vi "opencvDisplayImageTest.vi"() -> ()   [LabVIEW 2017]
uses:
  globalUtilities.vi
panel:
  out "x-y":dbl format="%.9f"
  in  "stop 4":bool
  out "Intensity Graph":u16[][](graph)
  in  "stop 3":bool
  # "Arrays work only if they have size >1 (2 is fine). Dunno why."
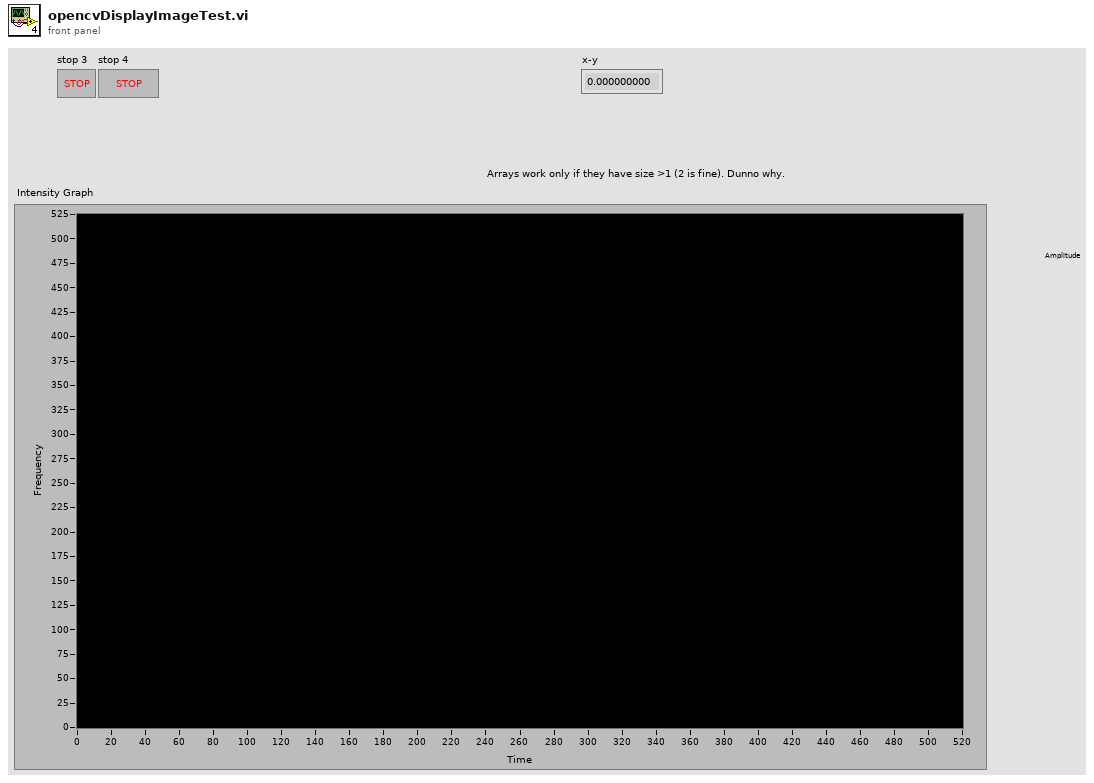
[diagram p1: front panel]
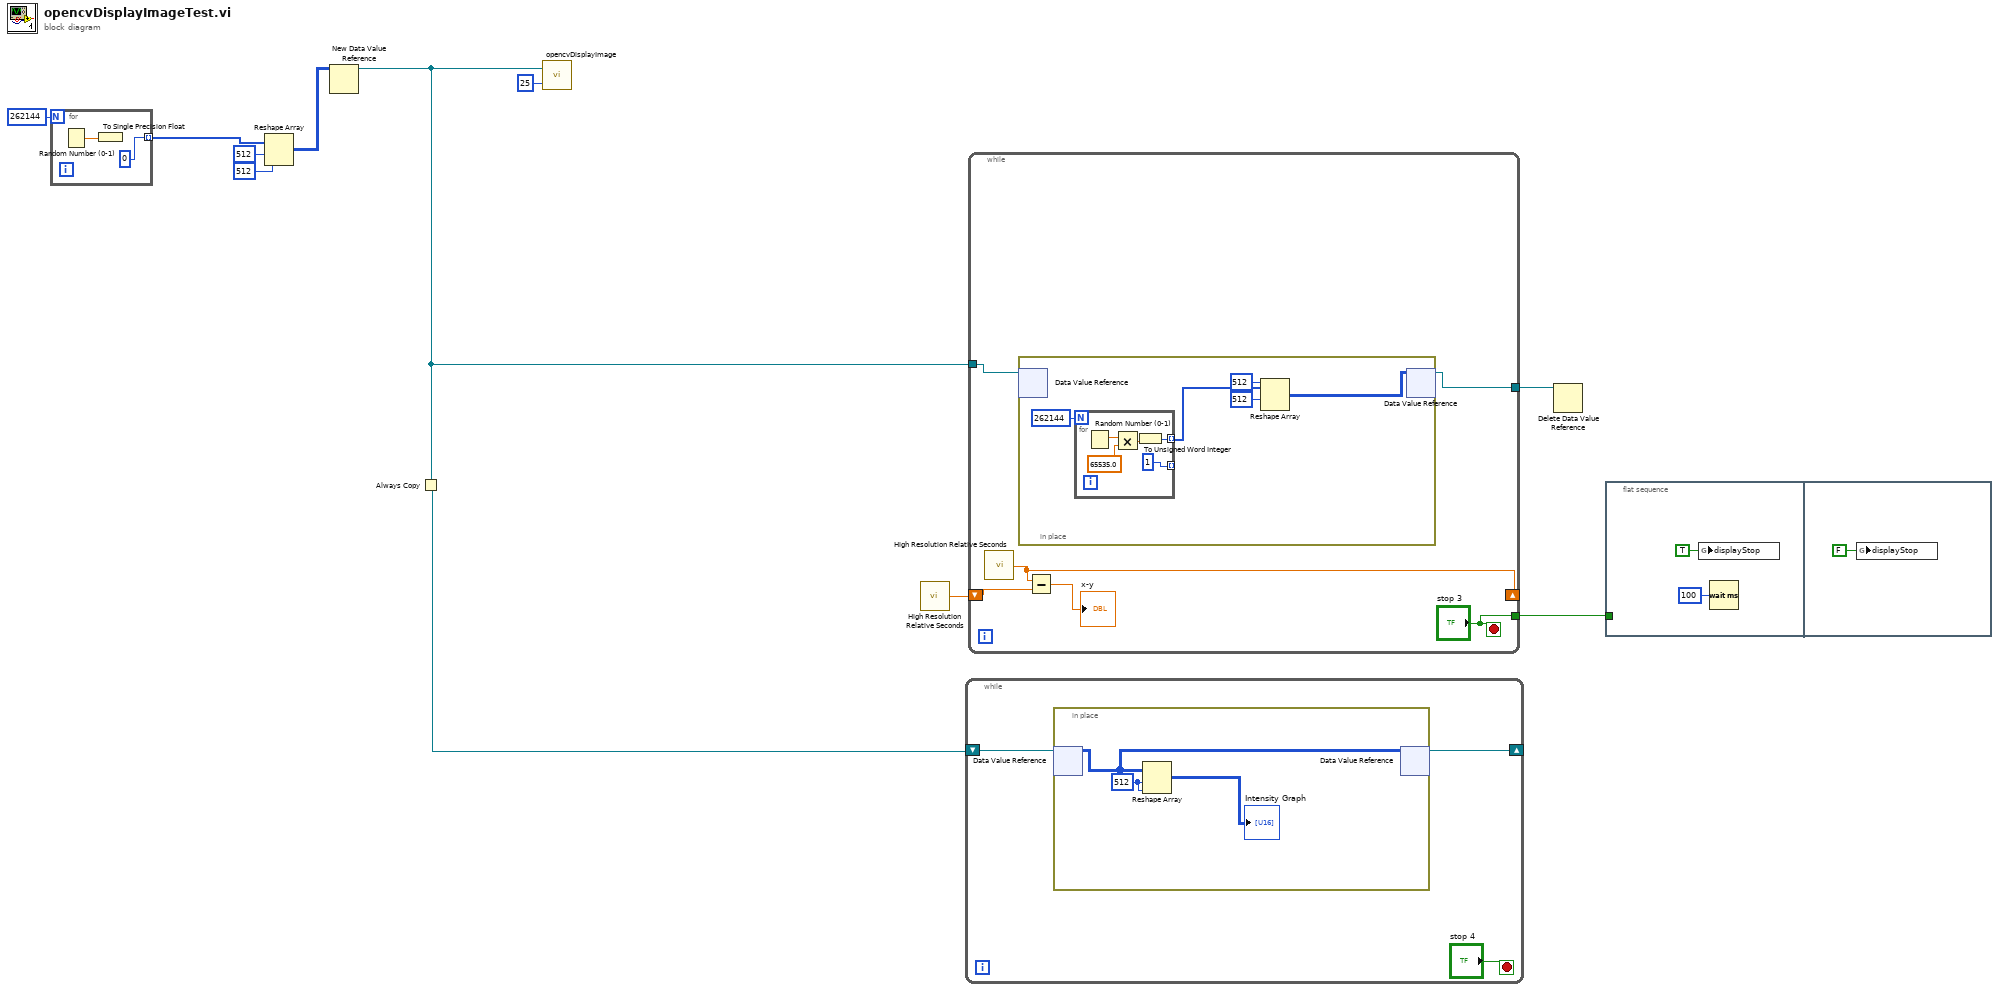
[diagram p0: block diagram]
diagram:
  n1 = for {
    N: 262144 ("dimension size") -> [_]
    tunnel: [u16 0] -> w5 mode=indexing
    n2 = Random Number (0-1)() -> (number: 0 to 1=w13:dbl)
    n3 = To Single Precision Float(number=w13) -> ()  [unwired: 1 out]
  }
  n4 = Reshape Array(w5, 512 ("dimension size"), 512 ("dimension size")) -> (w2:u16[][])
  n5 = New Data Value Reference(data value=w2) -> (data value reference=w7:refnum<data-value>)  [unwired: 1 in, 1 out]
  n6 = Always Copy(1:w7) -> (0:w9:refnum<data-value>)
  n7 = call "opencvDisplayImage.vi"("refresh_time"=25, "image reference"=w7) -> ()  [unwired: 1 in]
  n8 = call <vilib>:"High Resolution Relative Seconds.vi"() -> ("relative seconds"=w8:dbl)
  n9 = while {
    shift-right: [w15] -> _
    shift-left: w9 -> [w16]
    stop <- "stop 4" stop-if-true
    n10 = in-place {
      w19 = 512 ("dimension size")
      n11 = in-place-dvr #1(w16) -> (w17:u16[][])  [unwired: 1 out]
      n12 = Reshape Array(w17, w19, w19) -> (→"Intensity Graph":u16[][])
      n13 = in-place-dvr #1(w17) -> (w15:refnum<data-value>)  [unwired: 1 out]
    }
  }
  n14 = while {
    tunnel: w7 -> [w25]
    tunnel: [w24] -> w11
    shift-right: [w21] -> _
    shift-left: w8 -> [w23]
    tunnel: ["stop 3"] -> w1
    stop <- "stop 3" stop-if-true
    n15 = call <vilib>:"High Resolution Relative Seconds.vi"() -> ("relative seconds"=w21:dbl)
    n16 = in-place {
      n17 = in-place-dvr #2(w25) -> ()  [unwired: 2 out]
      n18 = for {
        N: 262144 ("dimension size") -> [_]
        tunnel: [w35] -> w29 mode=indexing
        tunnel: [u16 1] -> _ mode=indexing
        n19 = Random Number (0-1)() -> (number: 0 to 1=w33:dbl)
        n20 = Multiply(x=w33, y=65535.0) -> (x*y=w31:dbl)
        n21 = To Unsigned Word Integer(number=w31) -> (unsigned 16bit integer=w35:u16)
      }
      n22 = Reshape Array(w29, 512 ("dimension size"), 512 ("dimension size")) -> (w26:u16[][])
      n23 = in-place-dvr #2(w26) -> (w24:refnum<data-value>)  [unwired: 1 out]
    }
    n24 = Subtract(x=w21, y=w23) -> (x-y=→"x-y":dbl)
  }
  n25 = Delete Data Value Reference(data value reference=w11) -> ()  [unwired: 1 in, 2 out]
  n26 = flat-sequence {
    tunnel: w1 -> [_]
    frame #0 {
      n27 = global write "globalUtilities.vi" "displayStop"(TRUE ("generalStop")) -> ()
      n28 = Wait (ms)(milliseconds to wait=u32 100) -> ()  [unwired: 1 out]
    }
    frame #1 {
      n29 = global write "globalUtilities.vi" "displayStop"(FALSE ("generalStop")) -> ()
    }
  }
